vi "Main.vi"() -> ()   [LabVIEW 2017]
doc: "The myRIO Project template acquires acceleration data from the onboard accelerometer and displays the changes of acceleration values in a waveform chart."
uses:
  Coords Input Cluster.ctl
  Flow Control Enum.ctl
  <vilib>/myRIO/Instrument Drivers/Onboard IO/PWM/typedefs/PWM Reference.ctl
  <vilib>/myRIO/Common/Instrument Driver Framework/Utilities/typedefs/myRIO Generic Hardware Reference.ctl
  <vilib>/myRIO/Common/Instrument Driver Framework/Utilities/typedefs/Hardware Version Enum.ctl
  <vilib>/myRIO/Common/Instrument Driver Framework/Utilities/typedefs/myRIO v1.0 Reference.ctl
  <vilib>/myRIO/Common/Instrument Driver Framework/Utilities/typedefs/Generic FPGA Reference.ctl
  <vilib>/myRIO/Common/Instrument Driver Framework/myRIO v1.0/PWM/typedefs/PWM Channels Enum.ctl
  <vilib>/myRIO/Instrument Drivers/Onboard IO/PWM/typedefs/PWM Configuration.ctl
  <vilib>/userdefined/High Color/nirio_resource_hc.ctl
  <vilib>/myRIO/Common/Instrument Driver Framework/Utilities/vis/Is FPGA Ref Available.vi
  <vilib>/myRIO/Common/Instrument Driver Framework/myRIO v1.0/PWM/vis/myRIO v1.1 Open PWM.vi
  <vilib>/myRIO/Instrument Drivers/Onboard IO/PWM/vis/Set Duty Cycle and Frequency.vi
  <vilib>/myRIO/Common/Instrument Driver Framework/Utilities/vis/Validate Channels.vi
  <vilib>/myRIO/Common/Instrument Driver Framework/myRIO v1.0/PWM/vis/myRIO v1.0 Reserve PWM.vi
  <vilib>/myRIO/Common/Instrument Driver Framework/myRIO v1.0/UART/vis/myRIO v1.0 Close UART.vi
  <vilib>/myRIO/Common/Instrument Driver Framework/myRIO v1.0/PWM/vis/myRIO v1.0 Build MUX Configuration PWM.vi
  <vilib>/myRIO/Common/Instrument Driver Framework/myRIO v1.0/Resource Manager/vis/myRIO v1.0 Reserve Channel List.vi
  <vilib>/myRIO/Common/Instrument Driver Framework/myRIO v1.0/Resource Manager/vis/myRIO v1.0 Create Configuration List.vi
  <vilib>/myRIO/Common/Instrument Driver Framework/myRIO v1.0/Resource Manager/vis/myRIO v1.0 Reserve Channel.vi
  <vilib>/myRIO/Common/Instrument Driver Framework/myRIO v1.0/Resource Manager/vis/myRIO v1.0 Unreserve Channel.vi
  <vilib>/myRIO/Common/Instrument Driver Framework/myRIO v1.0/Resource Manager/vis/myRIO v1.0 Build Mutex Name.vi
  Vision Global Var..vi
  <vilib>/Utility/VariantDataType/GetNumericInfo.vi
  <vilib>/Utility/error.llb/Error Cluster From Error Code.vi
  <vilib>/myRIO/Common/Instrument Driver Framework/myRIO v1.0/myRIO v1.1 Open.vi
  <vilib>/myRIO/Common/Instrument Driver Framework/Utilities/vis/IO Manager.vi
  <vilib>/myRIO/Common/Instrument Driver Framework/Utilities/vis/Configuration Manager.vi
  <vilib>/myRIO/Common/Instrument Driver Framework/myRIO v1.0/Resource Manager/vis/myRIO v1.0 Configure IO.vi
  <vilib>/myRIO/Common/Instrument Driver Framework/myRIO v1.0/myRIO v1.0 Close.vi
  <vilib>/myRIO/Common/Instrument Driver Framework/myRIO v1.0/PWM/vis/myRIO v1.0 Write PWM.vi
  <vilib>/myRIO/Common/Instrument Driver Framework/Utilities/vis/FPGA Ref Manager.vi
  <vilib>/myRIO/Common/Instrument Driver Framework/myRIO v1.0/myRIO v1.0 Reset FPGA.vi
  <vilib>/myRIO/Common/Instrument Driver Framework/myRIO v1.0/IRQ/vis/myRIO v1.0 IRQ Info FGV.vi
  <vilib>/myRIO/Common/Instrument Driver Framework/myRIO v1.0/IRQ/vis/myRIO v1.0 Timer IRQ Info FGV.vi
  <vilib>/myRIO/Common/Instrument Driver Framework/myRIO v1.0/IRQ/vis/myRIO v1.0 ISR Agent.vi
  <vilib>/myRIO/Express VI/Onboard IO/PWM/PWM Express VI.xnode
  <vilib>/myRIO/Instrument Drivers/Onboard IO/PWM/vis/myRIO PWM Open.xnode
  <vilib>/myRIO/Instrument Drivers/Utilities/Utilities.lvlib
  <vilib>/myRIO/Instrument Drivers/Onboard IO/PWM/PWM.lvlib
panel:
  out "XY\nCompleted?":bool
  in  "Angle Tolerance (°)":dbl=0.5 format="%#_13g"
  out "Kicker Stepper \nON/OFF":bool
  out "Loop Counter":i32
  out "Solenoid\nON/OFF":bool
  out "Kicker Outputs":T1
  in  "Kicker Inputs":T2
  out "Y Acceleration":dbl[][](graph)
  out "Y Displacment":dbl[][](graph)
  out "Y Velocity":dbl[][](graph)
  in  "Y Axis Setpoint":T3
  in  "Coordinates Input":T4={"X-axis (mm)"=0.0, "Y-axis (mm)"=0.0, "Y dist  target \nthreshold (mm)"=1.0, "X dist target\nthreshold (mm)"=0.0} {"X dist target\nthreshold (mm)" min=0.0; "Y dist  target \nthreshold (mm)" min=0.0}
  out "Y Axis":T5(graph)
  out "X Axis":T5(graph)
  in  "X Axis Setpoint":T6
  in  "stop":bool
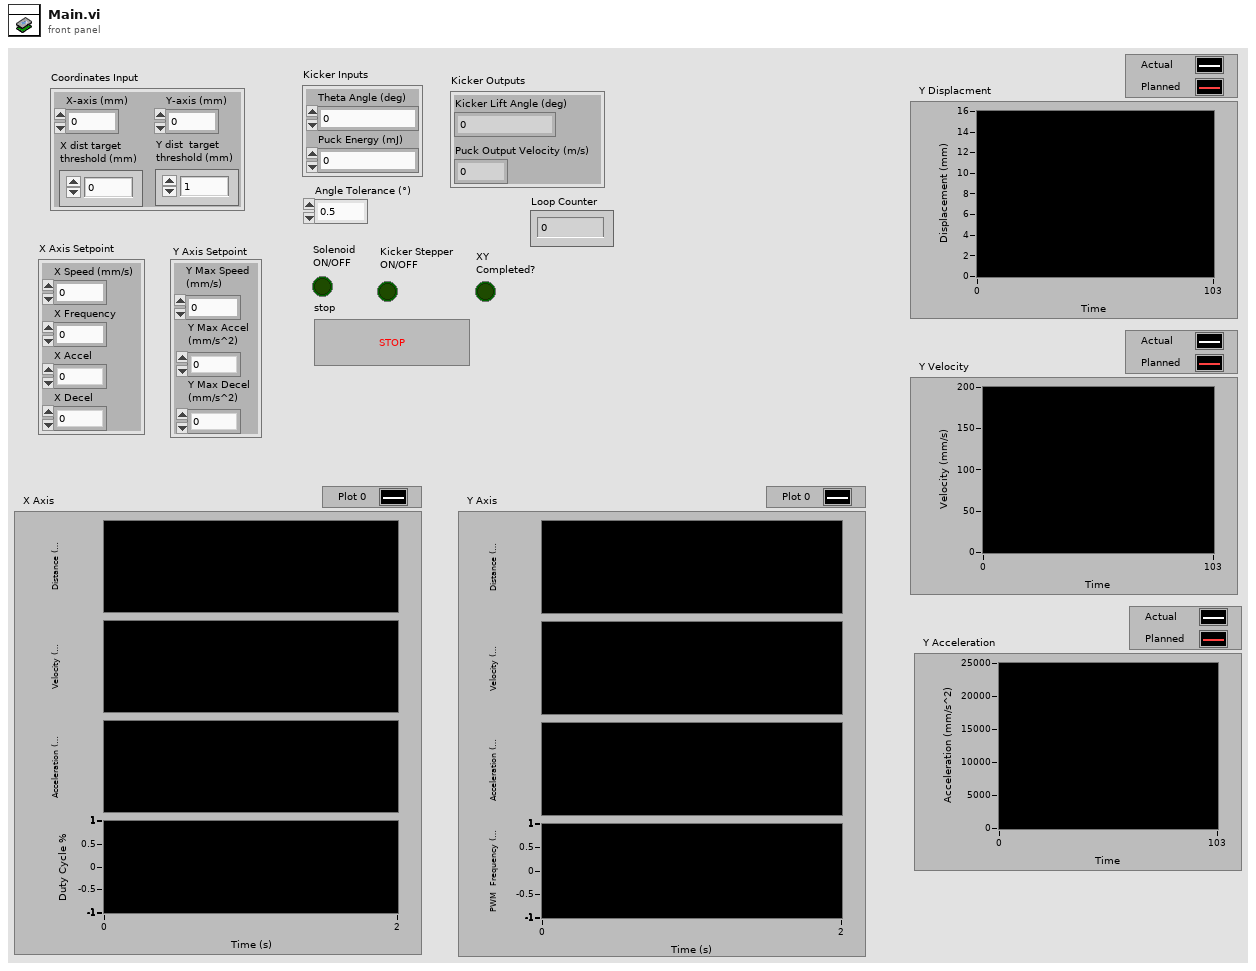
[diagram p1: front panel]
types:
  T1 = cluster{"Kicker Lift Angle (deg)":dbl, "Puck Output Velocity (m/s)":dbl}
  T2 = cluster{"Theta Angle (deg)":dbl, "Puck Energy (mJ)":dbl}
  T3 = cluster{"Y Max Speed \n(mm/s)":dbl, "Y Max Accel\n(mm/s^2)":dbl, "Y Max Decel \n(mm/s^2)":dbl}
  T4 = typedef "Coords Input Cluster.ctl" = cluster{"X-axis (mm)":dbl, "Y-axis (mm)":dbl, "Y dist  target \nthreshold (mm)":dbl, "X dist target\nthreshold (mm)":dbl}
  T5 = cluster{"X-axis distance":dbl, dbl, dbl, "X Frequency":dbl}
  T6 = cluster{"X Frequency":dbl, "X Accel":dbl, "X Decel":dbl, "X Speed (mm/s)":dbl}
  T7 = cluster{"X Axis Setpoint":cluster{"X Frequency":dbl, "X Accel":dbl, "X Decel":dbl, "X Speed (mm/s)":dbl}, "Y Axis Setpoint":cluster{"Y Max Speed \n(mm/s)":dbl, "Y Max Accel\n(mm/s^2)":dbl, "Y Max Decel \n(mm/s^2)":dbl}, "Y Velocity":dbl[][], "Y Displacment":dbl[][], "Y Acceleration":dbl[][], "X Axis":cluster{"X-axis distance":dbl, dbl, dbl, "X Frequency":dbl}, "Y Axis":cluster{"X-axis distance":dbl, dbl, dbl, "X Frequency":dbl}, "XY\nCompleted?":bool, "Coordinates Input ":T4, "Data Array":dbl[][]}
  T8 = cluster{"Kicker Inputs":cluster{"Theta Angle (deg)":dbl, "Puck Energy (mJ)":dbl}, "Kicker Outputs":cluster{"Kicker Lift Angle (deg)":dbl, "Puck Output Velocity (m/s)":dbl}, "Solenoid\nON/OFF":bool, "Kicker Stepper \nON/OFF":bool, "Angle Tolerance (°)":dbl, "Current Motor Step":i32}
  T9 = typedef "Flow Control Enum.ctl" = enum16{"Update I/O", "Kicker", "XY Drive", "Theta Axis", "Solenoid"}
  T10 = cluster{"Kicked?":bool, "Stop?":bool, "State":T9}
  T11 = cluster{"Y Velocity":dbl[][], "Y Displacment":dbl[][], "Y Acceleration":dbl[][]}
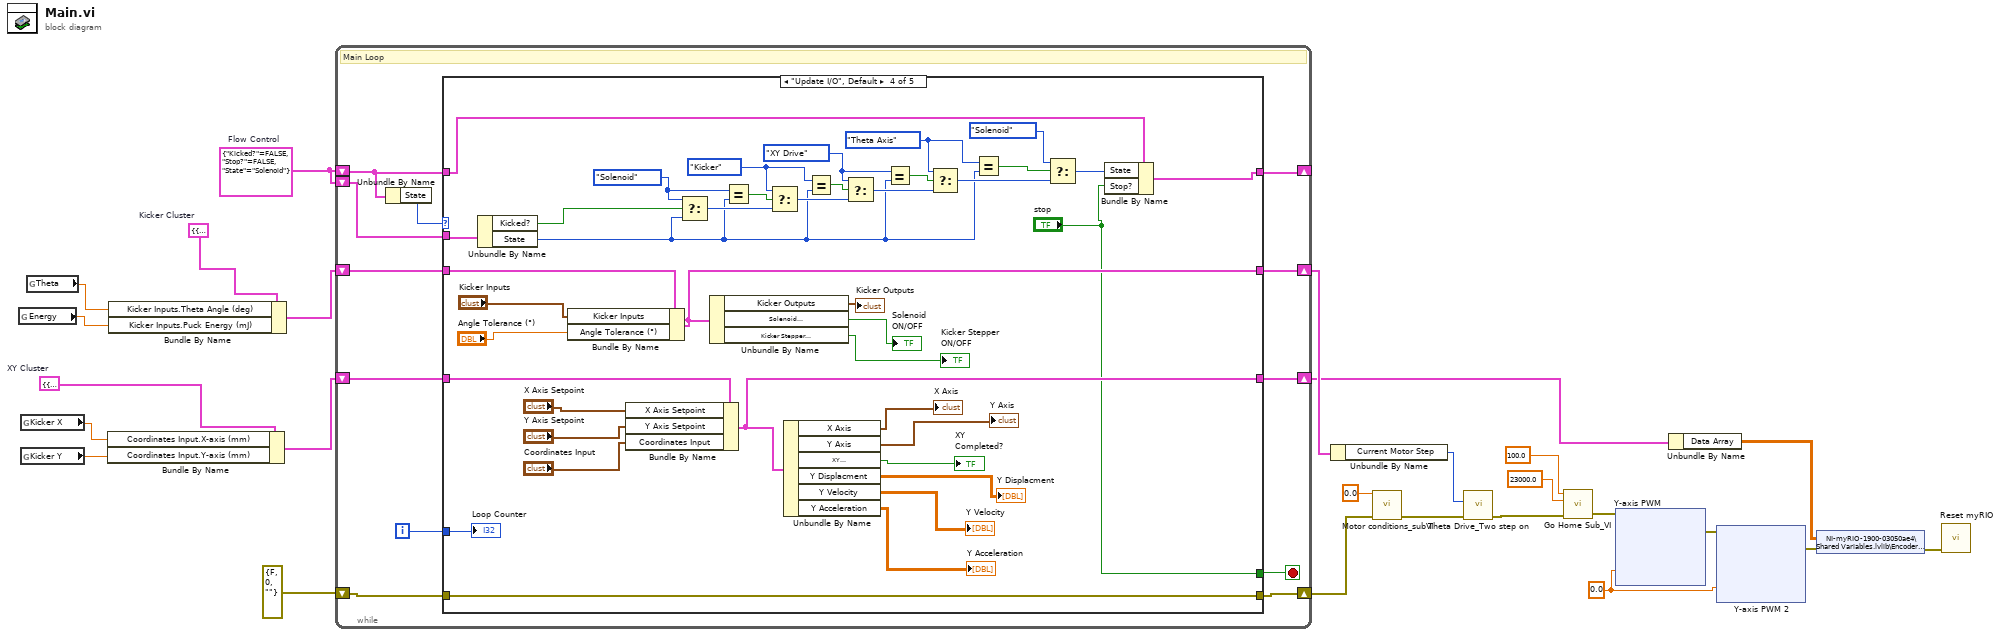
[diagram p0: block diagram]
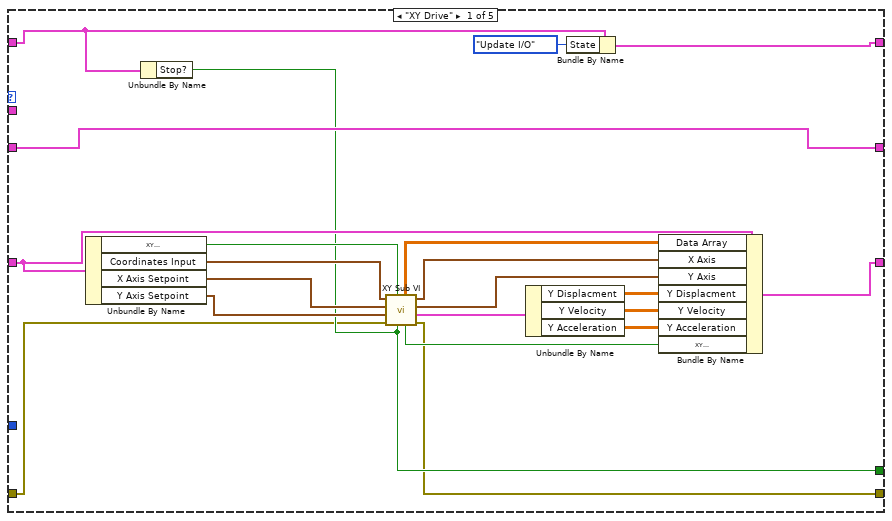
[diagram p2: hidden frame]
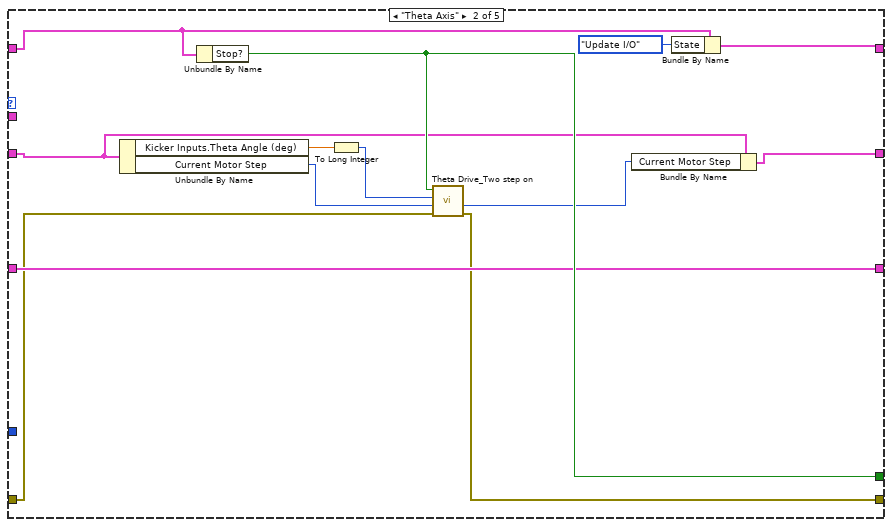
[diagram p3: hidden frame]
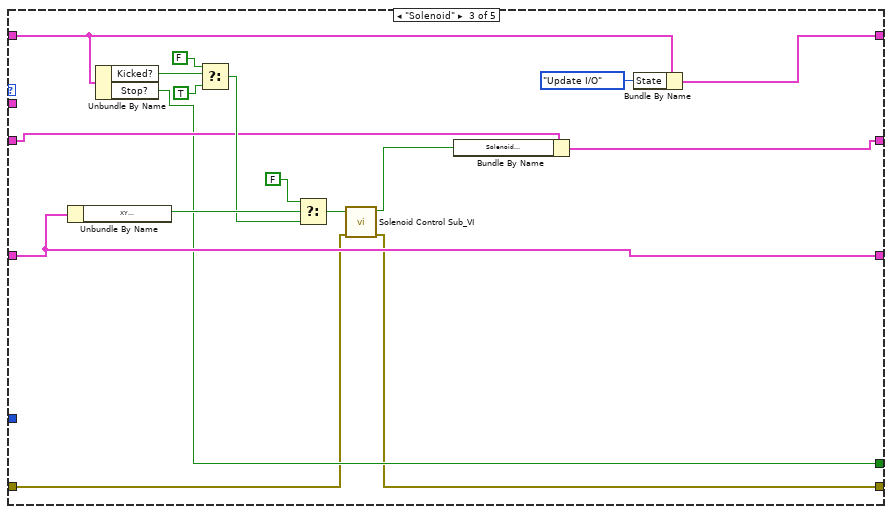
[diagram p4: hidden frame]
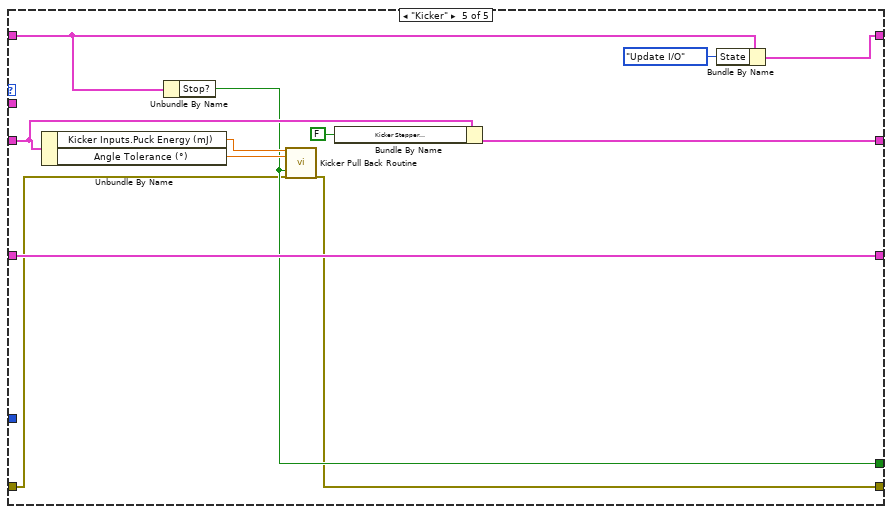
[diagram p5: hidden frame]
diagram:
  w4 = T7 {"X Axis Setpoint"={"X Frequency"=0.0, "X Accel"=0.0, "X Decel"=0.0, "X Speed (mm/s)"=0.0}, "Y Axis Setpoint"={"Y Max Speed \n(mm/s)"=0.0, "Y Max Accel\n(mm/s^2)"=0.0, "Y Max Decel \n(mm/s^2)"=0.0}, "Y Velocity"=[], "Y Displacment"=[], "Y Acceleration"=[], "X Axis"={"X-axis distance"=0.0, 0.0, 0.0, "X Frequency"=0.0}, "Y Axis"={"X-axis distance"=0.0, 0.0, 0.0, "X Frequency"=0.0}, "XY\nCompleted?"=FALSE, "Coordinates Input "={"X-axis (mm)"=0.0, "Y-axis (mm)"=0.0, "Y dist  target \nthreshold (mm)"=1.0, "X dist target\nthreshold (mm)"=0.0}, "Data Array"=[]}  # XY Cluster
  w8 = T8 {"Kicker Inputs"={"Theta Angle (deg)"=0.0, "Puck Energy (mJ)"=0.0}, "Kicker Outputs"={"Kicker Lift Angle (deg)"=0.0, "Puck Output Velocity (m/s)"=0.0}, "Solenoid\nON/OFF"=FALSE, "Kicker Stepper \nON/OFF"=FALSE, "Angle Tolerance (°)"=0.5, "Current Motor Step"=0}  # Kicker Cluster
  w9 = T10 {"Kicked?"=FALSE, "Stop?"=FALSE, "State"=enum."Solenoid"}  # Flow Control
  w21 = 0.0 ("Frequency [Hz]")
  n1 = global read "Vision Global Var..vi" "Energy"() -> (w5:dbl)
  n2 = global read "Vision Global Var..vi" "Kicker X"() -> (w3:dbl)
  n3 = global read "Vision Global Var..vi" "Kicker Y"() -> (w2:dbl)
  n4 = global read "Vision Global Var..vi" "Theta"() -> (w6:dbl)
  n5 = Bundle By Name(cluster=w4, "Coordinates Input.X-axis (mm)"=w3, "Coordinates Input.Y-axis (mm)"=w2) -> (w1:T7)
  n6 = Bundle By Name(cluster=w8, "Kicker Inputs.Theta Angle (deg)"=w6, "Kicker Inputs.Puck Energy (mJ)"=w5) -> (w7:T8)
  n7 = while {
    shift-right: [w27] -> w18
    shift-left: errorcluster {"status"=FALSE, "code"=0, "source"=""} ("error in (no error)") -> [w28]
    shift-right: [w34] -> _
    shift-left: w9 -> [w37]
    shift-right: [w29] -> w11
    shift-left: w1 -> [w32]
    shift-right: [w30] -> w12
    shift-left: w7 -> [w31]
    shift-left: w9 -> [w26]
    i -> [w33]
    stop <- w35 stop-if-true
    # "Main Loop"
    n8 = Unbundle By Name(w37) -> ("State"=w36:T9)
    n9 = case shown="\"Update I/O\", Default" w36 {
      tunnel: w37 -> [w42 w69 w77 w96 w134]
      tunnel: [w41 w68 w74 "stop" w132] -> w35
      tunnel: [w57 w70 w76 w95 w140] -> w34
      tunnel: w33 -> [_ _ _ w128 _]
      tunnel: w32 -> [w55 w61 w78 w111 w133]
      tunnel: w31 -> [w56 w64 w81 w113 w136]
      tunnel: [w56 w63 w80 w112 w135] -> w30
      tunnel: [w54 w61 w78 w110 w133] -> w29
      tunnel: w28 -> [w39 w60 w73 w92 w131]
      tunnel: [w38 w59 w72 w92 w130] -> w27
      tunnel: w26 -> [_ _ _ w91 _]
      frame "XY Drive" {
        n10 = Unbundle By Name(w55) -> ("XY\nCompleted?"=w43:bool, "Coordinates Input"=w53:T4, "X Axis Setpoint"=w52:T6, "Y Axis Setpoint"=w51:T3)
        n11 = Unbundle By Name(w42) -> ("Stop?"=w41:bool)
        n12 = call "XY Sub VI.vi"("stop"=w41, "Movement\nComplete?"=w43, "error in (no error)"=w39, "Y Axis Setpoint"=w51, "X Axis Setpoint"=w52, "Coordinates Input"=w53) -> ("error out"=w38:errorcluster, "Y Path Display"=w48:T11, "Y Axis"=w49:T5, "X Axis"=w50:T5, "Completed?"=w44:bool, "Data Array"=w40:dbl[][])
        n13 = Unbundle By Name(w48) -> ("Y Displacment"=w47:dbl[][], "Y Velocity"=w46:dbl[][], "Y Acceleration"=w45:dbl[][])
        n14 = Bundle By Name(cluster=w42, "State"=Flow_Control_Enum."Update I/O") -> (w57:T10)
        n15 = Bundle By Name(cluster=w55, "Data Array"=w40, "X Axis"=w50, "Y Axis"=w49, "Y Displacment"=w47, "Y Velocity"=w46, "Y Acceleration"=w45, "XY\nCompleted?"=w44) -> (w54:T7)
      }
      frame "Theta Axis" {
        n16 = Unbundle By Name(w64) -> ("Kicker Inputs.Theta Angle (deg)"=w67:dbl, "Current Motor Step"=w65:i32)
        n17 = Unbundle By Name(w69) -> ("Stop?"=w68:bool)
        n18 = To Long Integer(number=w67) -> (32bit integer=w66:i32)
        n19 = call "Theta Drive_Two step on.vi"("error in (no error)"=w60, "Start Location Step (-90to90)"=w65, "Target Step (-90to90)"=w66, "stop"=w68) -> ("error out"=w59:errorcluster, "Current Motor Step (0to3)"=w62:i32)  [unwired: 4 in, 2 out]
        n20 = Bundle By Name(cluster=w64, "Current Motor Step"=w62) -> (w63:T8)
        n21 = Bundle By Name(cluster=w69, "State"=Flow_Control_Enum."Update I/O") -> (w70:T10)
      }
      frame "Solenoid" {
        n22 = Unbundle By Name(w78) -> ("XY\nCompleted?"=w85:bool)
        n23 = Unbundle By Name(w77) -> ("Kicked?"=w88:bool, "Stop?"=w74:bool)
        n24 = Select(t=FALSE, s=w88, f=TRUE) -> (s? t:f=w83:bool)
        n25 = Select(t=FALSE, s=w85, f=w83) -> (s? t:f=w82:bool)
        n26 = call "Solenoid Control Sub_VI.vi"("error in (no error)"=w73, "SOLENOID ON/OFF"=w82) -> ("error out"=w72:errorcluster, "ON/OFF"=w79:bool)  [unwired: 8 in]
        n27 = Bundle By Name(cluster=w81, "Solenoid\nON/OFF"=w79) -> (w80:T8)
        n28 = Bundle By Name(cluster=w77, "State"=Flow_Control_Enum."Update I/O") -> (w76:T10)
      }
      frame "Update I/O", Default {
        w102 = Flow_Control_Enum."Theta Axis" ("State")
        w105 = Flow_Control_Enum."XY Drive" ("State")
        w106 = Flow_Control_Enum."Kicker" ("State")
        w107 = Flow_Control_Enum."Solenoid" ("State")
        n29 = Unbundle By Name(w91) -> ("Kicked?"=w90:bool, "State"=w89:T9)
        n30 = Bundle By Name(cluster=w113, "Kicker Inputs"="Kicker Inputs", "Angle Tolerance (°)"="Angle Tolerance (°)") -> (w112:T8)
        n31 = Bundle By Name(cluster=w111, "X Axis Setpoint"="X Axis Setpoint", "Y Axis Setpoint"="Y Axis Setpoint", "Coordinates Input"="Coordinates Input") -> (w110:T7)
        n32 = Select(t=w107, s=w90, f=w89) -> (s? t:f=w108:T9)
        n33 = Unbundle By Name(w112) -> ("Kicker Outputs"=→"Kicker Outputs":T1, "Solenoid\nON/OFF"=→"Solenoid\nON/OFF":bool, "Kicker Stepper \nON/OFF"=→"Kicker Stepper \nON/OFF":bool)
        n34 = Equal?(x=w107, y=w89) -> (x = y?=w109:bool)
        n35 = Select(t=w106, s=w109, f=w108) -> (s? t:f=w103:T9)
        n36 = Unbundle By Name(w110) -> ("X Axis"=→"X Axis":T5, "Y Axis"=→"Y Axis":T5, "XY\nCompleted?"=→"XY\nCompleted?":bool, "Y Displacment"=→"Y Displacment":dbl[][], "Y Velocity"=→"Y Velocity":dbl[][], "Y Acceleration"=→"Y Acceleration":dbl[][])
        n37 = Equal?(x=w106, y=w89) -> (x = y?=w104:bool)
        n38 = Select(t=w105, s=w104, f=w103) -> (s? t:f=w100:T9)
        n39 = Equal?(x=w105, y=w89) -> (x = y?=w101:bool)
        n40 = Select(t=w102, s=w101, f=w100) -> (s? t:f=w97:T9)
        n41 = Equal?(x=w102, y=w89) -> (x = y?=w98:bool)
        n42 = Select(t=Flow_Control_Enum."Solenoid" ("State"), s=w98, f=w97) -> (s? t:f=w94:T9)
        n43 = Bundle By Name(cluster=w96, "State"=w94, "Stop?"="stop") -> (w95:T10)
        "Loop Counter" <- w128
      }
      frame "Kicker" {
        n44 = Unbundle By Name(w136) -> ("Kicker Inputs.Puck Energy (mJ)"=w138:dbl, "Angle Tolerance (°)"=w137:dbl)
        n45 = Unbundle By Name(w134) -> ("Stop?"=w132:bool)
        n46 = call "Kicker Pull Back Routine.vi"("Puck Energy Requirement (mJ)"=w138, "Angle Tolerance (°)"=w137, "stop"=w132, "error in (no error)"=w131) -> ("error out"=w130:errorcluster)  [unwired: 13 in, 2 out]
        n47 = Bundle By Name(cluster=w136, "Kicker Stepper \nON/OFF"=FALSE ("Kicker Stepper \nON/OFF")) -> (w135:T8)
        n48 = Bundle By Name(cluster=w134, "State"=Flow_Control_Enum."Update I/O") -> (w140:T10)
      }
    }
  }
  n49 = Unbundle By Name(w12) -> ("Current Motor Step"=w13:i32)
  n50 = call "Motor conditions_subVI.vi"("Target Angle (°)"=0.0, "error in (no error)"=w18) -> ("error out"=w17:errorcluster)  [unwired: 11 in, 2 out]
  n51 = call "Theta Drive_Two step on.vi"("error in (no error)"=w17, "Target Step (-90to90)"=w13) -> ("error out"=w16:errorcluster)  [unwired: 6 in, 3 out]
  n52 = call "Go Home Sub_VI.vi"("error in (no error)"=w16, "Homing Freq"=23000.0, "Homing Duty %"=100.0) -> ("error out"=w14:errorcluster)  [unwired: 7 in, 1 out]
  n53 = xnode "Y-axis PWM"("Frequency [Hz]"=w21, "error in (no error)"=w14) -> ("error out"=w23:errorcluster)
  n54 = Unbundle By Name(w11) -> ("Data Array"=w10:dbl[][])
  n55 = xnode "Y-axis PWM 2"("Frequency [Hz]"=w21, "error in (no error)"=w23) -> ("error out"=w22:errorcluster)
  n56 = shared-variable "NI-myRIO-1900-03050ae4\\Shared Variables.lvlib\\Encoder Data"(w10, error in=w22) -> (error out=w24:errorcluster)
  n57 = call <vilib>:"Reset myRIO.vi"("error in (no error)"=w24) -> ()  [unwired: 10 in, 1 out]
